vi "Plate Tank 4.vi"() -> ()   [LabVIEW 2019]
uses:
  <vilib>/NI/Current Value Table/Type Defs/Single Tag.ctl
  <vilib>/NI/Current Value Table/Type Defs/Data Types.ctl
  <vilib>/Utility/sysdir.llb/System Directory Type.ctl
  <vilib>/NI/STM/TCP/Read Meta Data (TCP Ref).vi
  <vilib>/NI/STM/TCP/Get Connection Reference (TCP).vi
  <vilib>/NI/AMC/Read Termination Message.vi
  <vilib>/NI/AMC/Create Single Message.vi
  <vilib>/NI/AMC/Update Message Routing Info.vi
  <vilib>/NI/STM/TCP/Read Meta Data (TCP Clst).vi
  <vilib>/NI/AMC/Send Message.vi
  <vilib>/NI/AMC/Globals.vi
  <userlib>/_OpenG.lib/comparison/comparison.llb/I32 Changed__ogtk.vi
  <vilib>/NI/STM/TCP/Write Message (TCP).vi
  <vilib>/NI/AMC/AMC.lvlib
  <vilib>/NI/STM/NI STM.lvlib
  <vilib>/NI/Current Value Table/Current Value Table.lvlib
panel:
  in  "EZ Recipe Button":bool
  out "Loaded Recipe":string
  in  "Load A Recipe":bool
  in  "Save this Recipe":bool
  out "Right Time":dbl format="%.1f"
  out "Left Time":dbl format="%.1f"
  out "Total Amp*min R":dbl format="%.1f"
  out "Total Amp*min L":dbl format="%.1f"
  in  "Rectifer Settings":i32(listbox)
  in  "MO":string
  in  "BasT1_P Last Hr":bool
  in  "BasT1_Level Last Hr":bool
  out "Boolean 5":bool
  out "SumpBottom":bool
  out "Process 1 Supply":bool
  out "Sump Return":bool
  out "Boolean 2":bool
  out "SG":dbl format="%.3g"
  out "Return to sump 4":bool
  in  "Rectifer Data":enum32{"Standard", "Eng"}(tab)
  out "Current Step":i32
  out "Left Anode Actual Current":dbl(knob) scale=0.0..150.0
  out "Right Anode Actual Current":dbl(knob) scale=0.0..150.0
  out "Left Anode Amp-min":dbl(slide)
  out "Right Anode Amp-min":dbl(slide)
  out "Output Voltage":cluster{dbl, dbl}(graph)
  in  "Tab Control 2":enum32{"Standard", "ENG"}(tab)
  out "Supply Flow":dbl(knob) scale=0.0..65.0
  out "Plating Cell Liquid Level":dbl(slide) scale=0.0..75.0
  out "Cell Temperature":dbl(slide) scale=0.0..60.0
  in  "Cell T Last Hr":bool
  out "Suck Pump":bool
  out "Suck Pump Flow":dbl format="%#_4g"
  out "SuckPipe":bool
  out "SuckPipe 3":bool
  out "Drain Tee Top":bool
  out "Return to sump 2":bool
  out "Return to sump 3":bool
  out "Flow Controller":dbl(knob) scale=0.0..100.0
  in  "Tab Control":enum32{"Main Pump", "Suck Pump"}(tab)
  out "Amps":dbl format="%#.2g"
  out "Volts":dbl format="%#.1f"
  out "VFD T":dbl format="%#.2g"
  out "RPM":dbl format="%#.0f"
  out "Fault Code":dbl format="%#.2g"
  out "Freq":dbl format="%#.2g"
  out "SP1 Amps":dbl caption="Amps" format="%#.2g"
  out "SP1 Volts":dbl caption="Volts" format="%#.1g"
  out "SP1 RPM":dbl caption="RPM" format="%#.2g"
  out "SP1 VFD T":dbl caption="VFD T" format="%#.2g"
  out "SP1 Fault Code":dbl caption="Fault Code" format="%#.2g"
  out "SP1 Freq":dbl caption="Freq" format="%#.2g"
  out "Flow 1":dbl format="%#_4g"
  out "Flow 2":dbl format="%#_4g"
  out "Flow 3":dbl format="%#_4g"
  out "Flow 4":dbl format="%#_4g"
  out "Return to sump":bool
  out "E Stop":bool
  out "Run Enabled?":bool
  in  "Full Drain Plating Cell":bool
  out "Rack Motion":bool
  out "Right Eductor Motion":bool
  out "Left Eductor Motion":bool
  out "Right Output On":bool
  in  "Enable Rack Motion":bool
  in  "Rack RPM":dbl(knob) scale=0.0..15.0
  out "Left Output On":bool
  in  "Start Cycle":bool
  in  "Cancel Cycle":bool
  out "SuckPipe 2":bool
  out "Main Pump":bool
  in  "Enable Eductor Motion":bool
  in  "Eductor RPM":dbl(knob) scale=0.0..15.0
  in  "Supply Pressure (kPa)":dbl(knob)=50.0 min=50.0 max=200.0 step=5.0 scale=50.0..200.0
  in  "Total Inflow (L/min)":dbl(knob)=40.0 min=25.0 max=50.0 step=0.5 scale=25.0..50.0
  in  "Suck Pump fraction of inflow":dbl(knob)=5.0 min=5.0 max=90.0 step=1.0 scale=0.0..90.0
  out "Sump Level":dbl(slide) scale=0.0..1000.0
  out "Supply Pressure":dbl(knob) scale=0.0..200.0
  in  "Enable Suck Pump":bool
  in  "Enable Plating Cell":bool
  in  "Machine":bool
  in  "Basement 4":bool
  in  "Dryer":bool
  in  "Rinse 4":bool
  in  "Rinse 3":bool
  in  "Rinse 2":bool
  in  "Basement 3":bool
  in  "Basement 2":bool
  in  "Basement 1":bool
  in  "Plater 6":bool
  in  "Plater 5":bool
  in  "Plater 4":bool
  in  "Plater 3":bool
  in  "Plater 2":bool
  in  "Plater 1":bool
  in  "Predip":bool
  in  "Rinse 1":bool
  in  "Cleaner":bool
  in  "Etch":bool
  out "status":string
  out "Boolean 4":bool
  # "Module Selection"
  # "Rectifier Settings"
  # "Recipe"
  # "Fluid Flow Control"
  # "Rectifier Control"
  # "Rectifier Output"
  # "Motion starts when rectifiers cycle"
  # "Note: RPM settings shared with tank 4"
  # "kPa"
  # "@"
  # "Output"
  # "cm"
  # "°C"
  # "L/min"
  # "cm"
  # "L/min"
  # "L/min"
  # "L/min"
  # "L/min"
  # "L/min"
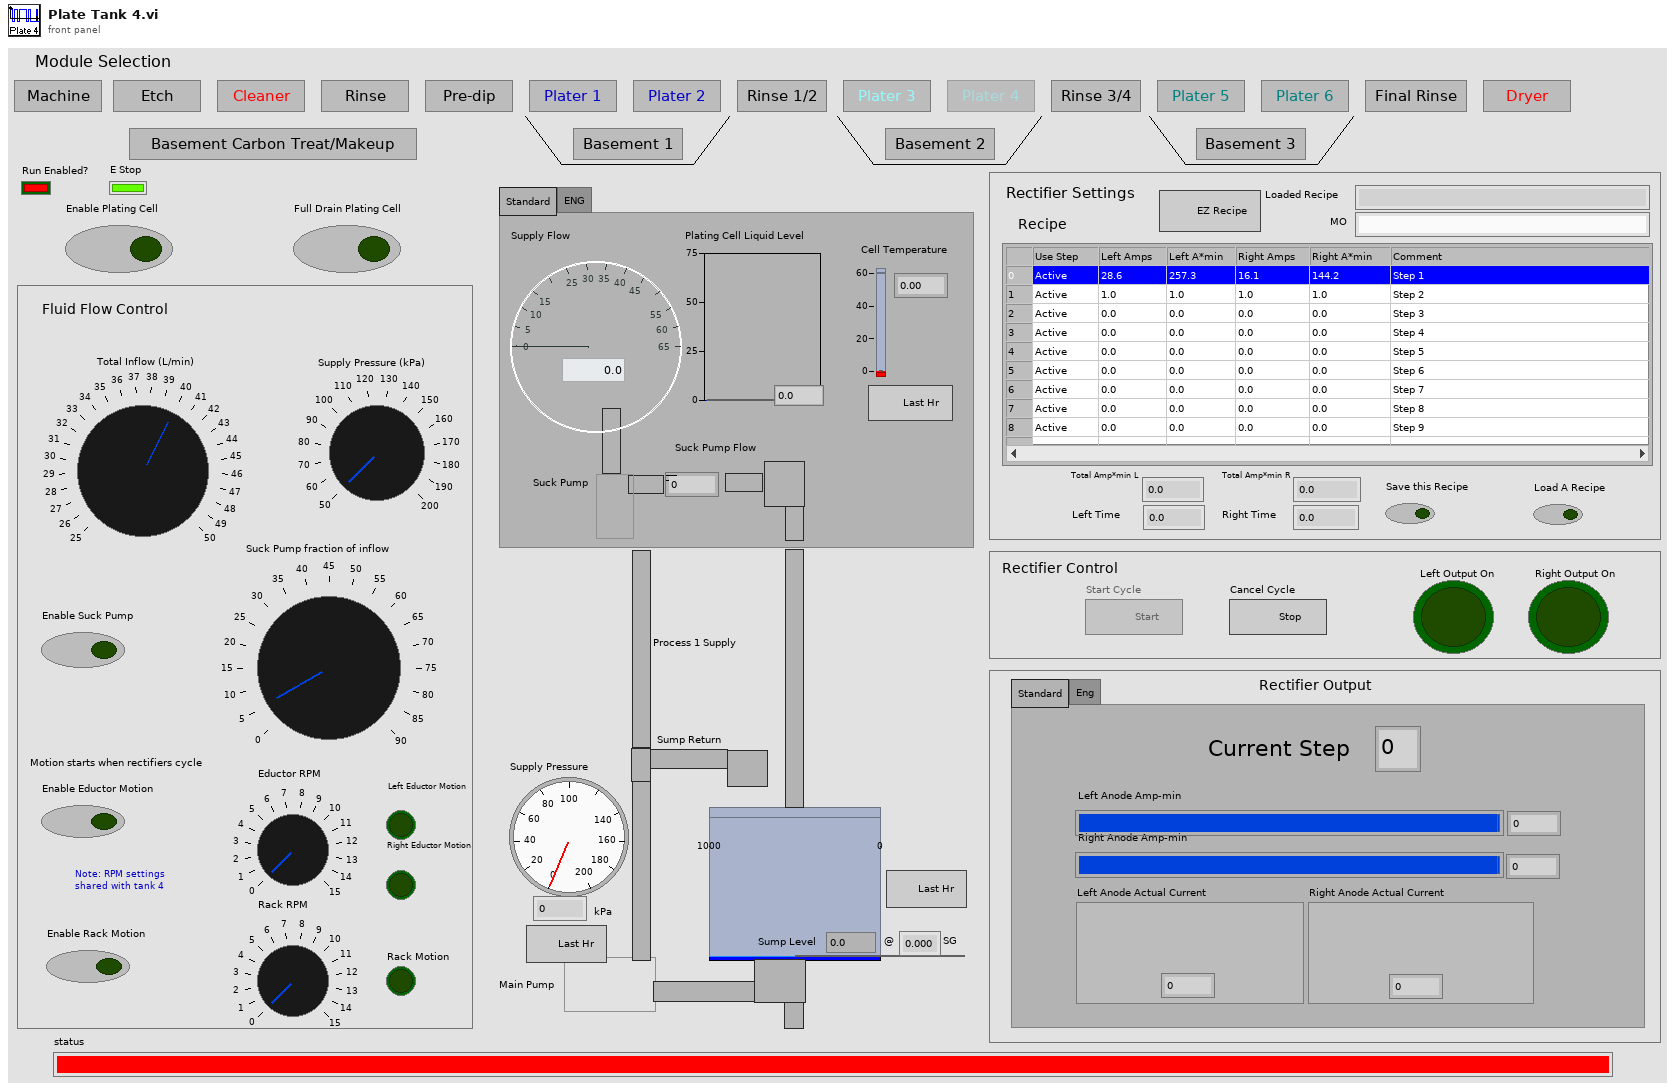
[diagram p1: front panel]
types:
  T1 = typedef "Current Value Table.lvlib/Single Tag.ctl" = cluster{"Data Type":T2, "Name":string, "Value":string, "Description":string}
  T2 = typedef "Current Value Table.lvlib/Data Types.ctl" = enum16{"Double", "Single", "I64", "I32", "I16", "I8", "U64", "U32", "U16", "U8", "String", "Boolean", "Array of U8", "Array of U16", "Array of U32", "Array of U64", "Array of I64", "Array of I32", "Array of I16", "Array of I8", "Array of Double", "Array of Single", "Array of Boolean", "Array of String"}
  T3 = typedef "NI STM.lvlib/TCP Connection Info.ctl" = cluster{"connection ID":refnum<k5>, "meta data":T4[]}
  T4 = typedef "NI STM.lvlib/MetaDataElement.ctl" = string
  T5 = typedef "AMC.lvlib/Message Queue.ctl" = refnum<queue>
  T6 = cluster{"Shift":bool, "Ctrl":bool, "Alt":bool, "Cmd":bool, "Opt":bool}
  T7 = typedef "LVPoint32TypeDef.ctl" = cluster{"Horizontal":i32, "Vertical":i32}
  T8 = typedef "LVRowAndColumnTypeDef.ctl" = cluster{"Row":i32, "Column":i32}
  T9 = enum8{"Enabled", "Disabled", "Disabled and Grayed Out"}
  T10 = typedef "System Directory Type.ctl" = i32
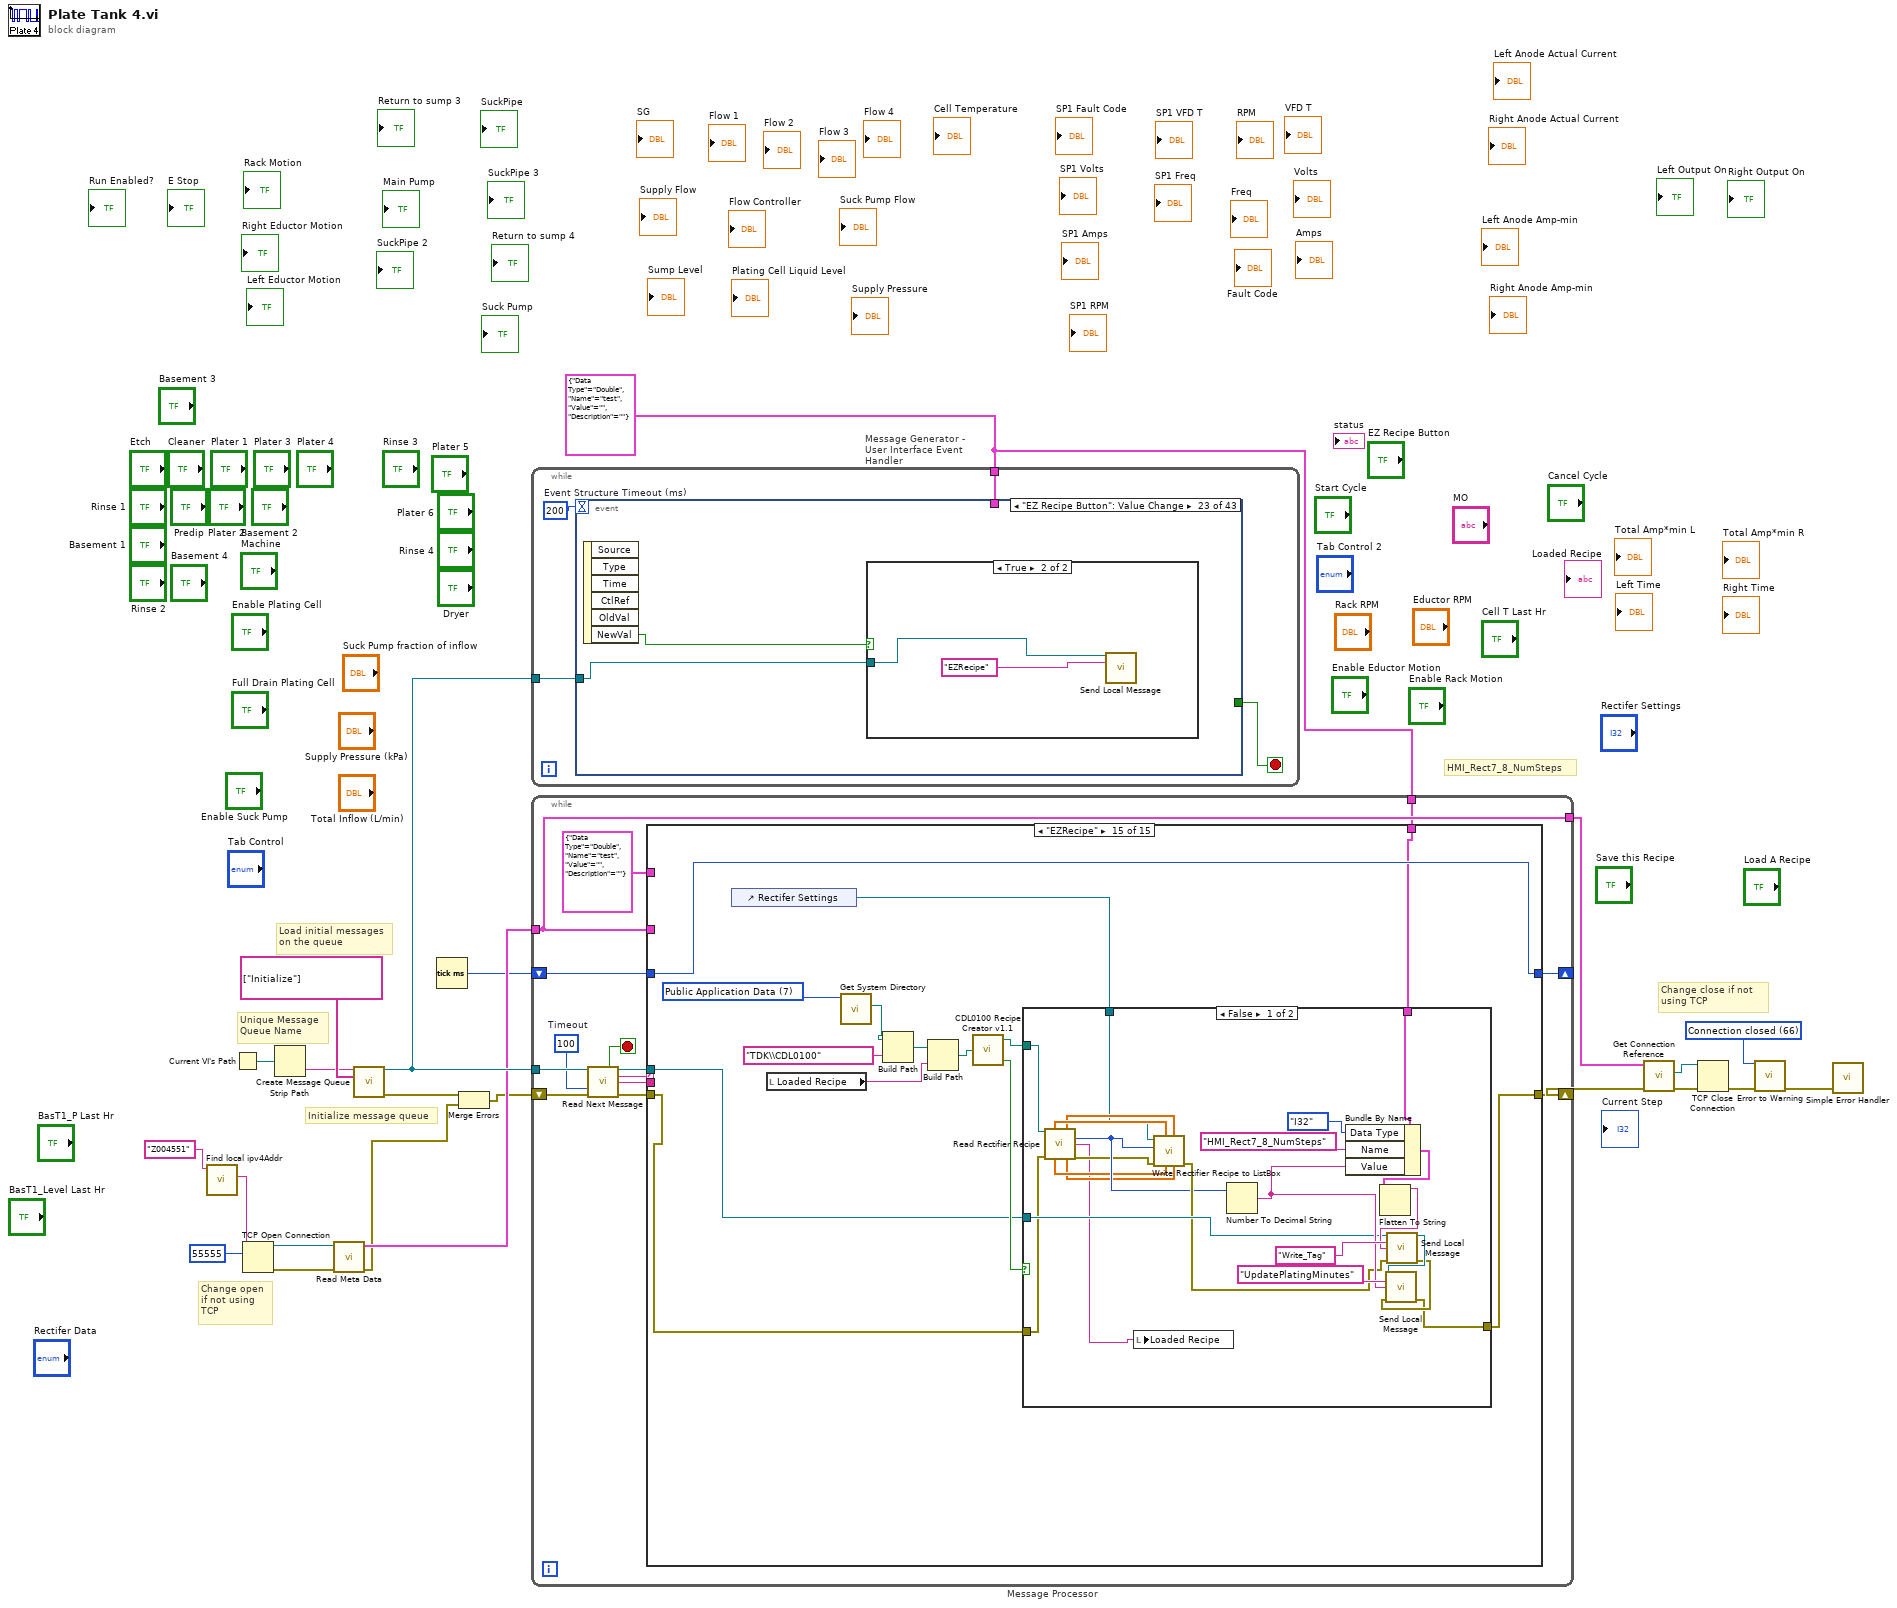
[diagram p0: block diagram]
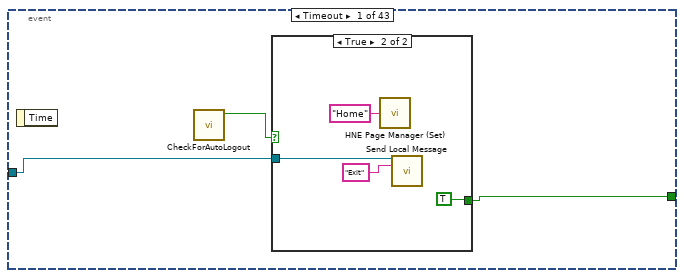
[diagram p2: hidden frame]
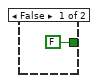
[diagram p3: hidden frame]
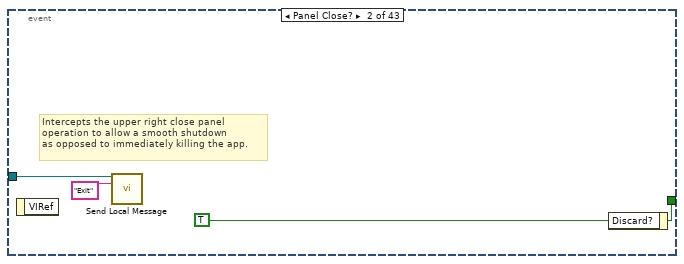
[diagram p4: hidden frame]
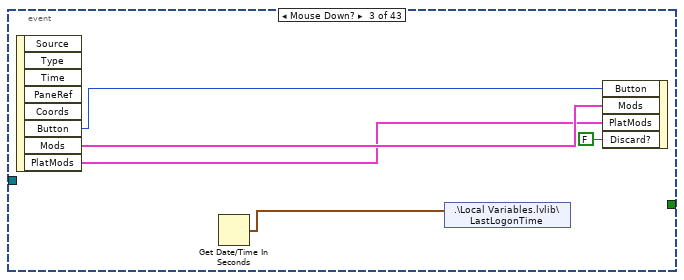
[diagram p5: hidden frame]
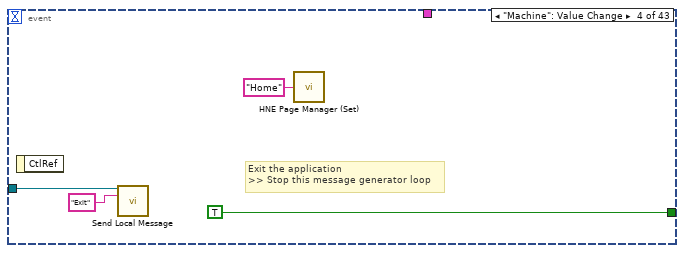
[diagram p6: hidden frame]
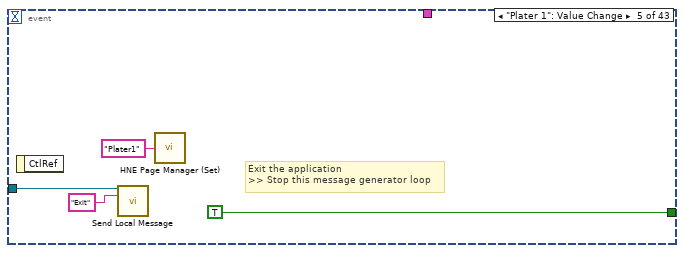
[diagram p7: hidden frame]
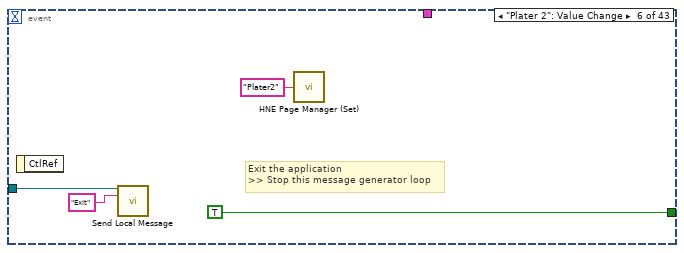
[diagram p8: hidden frame]
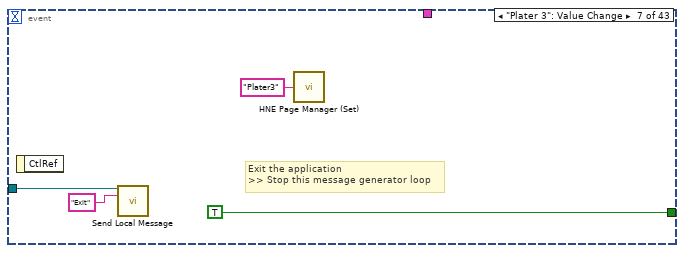
[diagram p9: hidden frame]
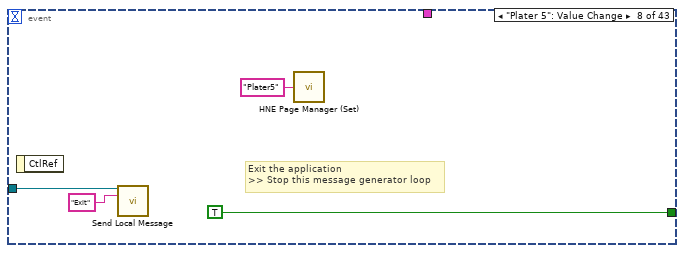
[diagram p10: hidden frame]
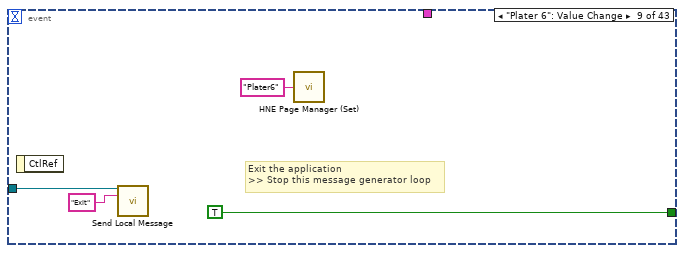
[diagram p11: hidden frame]
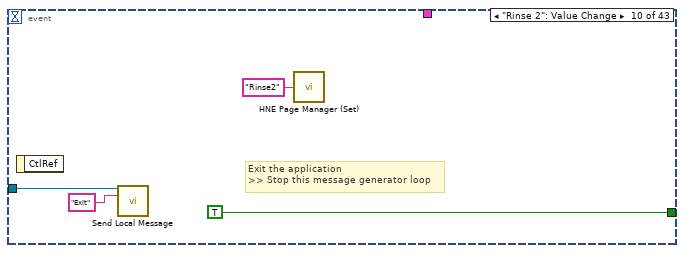
[diagram p12: hidden frame]
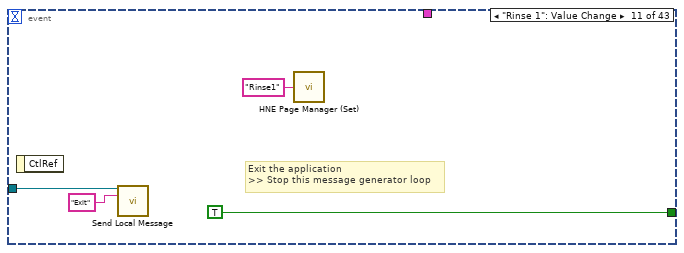
[diagram p13: hidden frame]
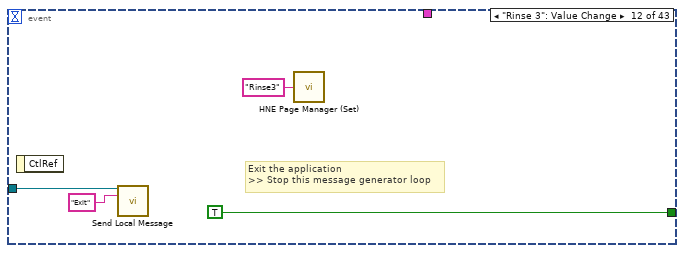
[diagram p14: hidden frame]
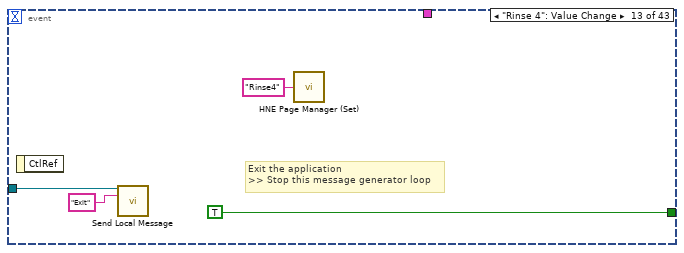
[diagram p15: hidden frame]
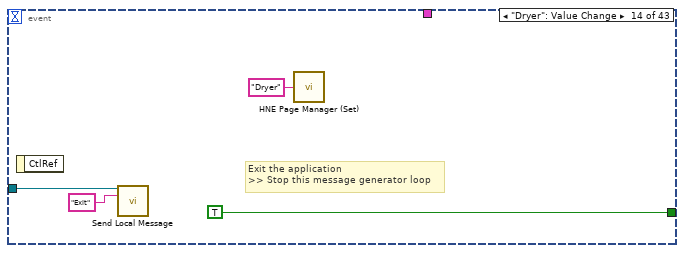
[diagram p16: hidden frame]
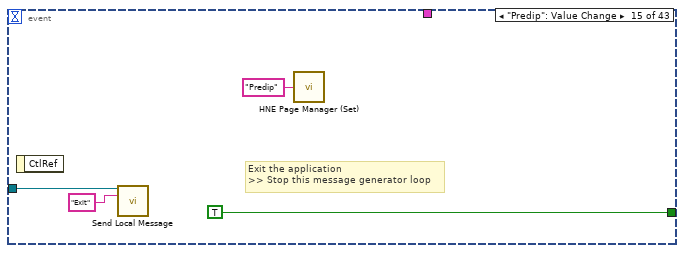
[diagram p17: hidden frame]
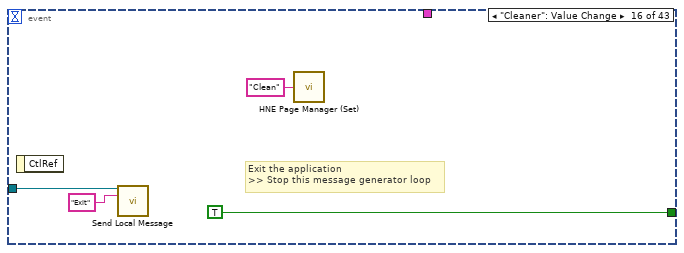
[diagram p18: hidden frame]
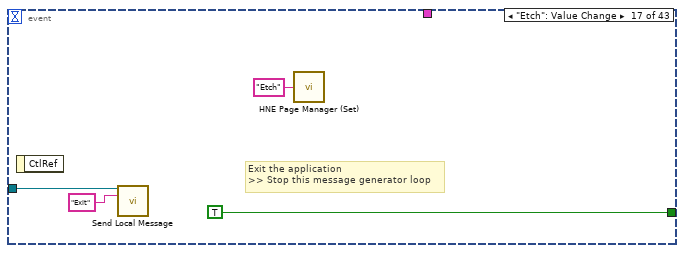
[diagram p19: hidden frame]
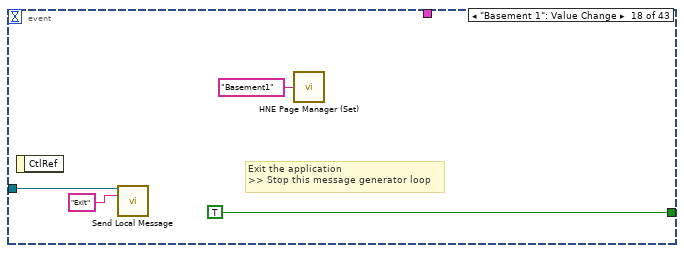
[diagram p20: hidden frame]
diagram:
  w1 = T1 {"Data Type"=enum."Double", "Name"="test", "Value"="", "Description"=""} ("Tag")
  w13 = 66 items=["No Error", "Argument Error", "Memory Full", "Out of Zone", "End of File", "File Already Open", "Generic File IO Error", "File Not Found", "File Permission Error", "Disk Full", "Duplicate Path", "Too Many Files Open", "Not Enabled", "Resource File Not Found", "Cannot Add Resource", "Resource Not Found", "Image Not Found", "Image Memory Error", "Pen Does Not Exist", "Config Bad Type", "Config Token Not Found", "Config Parse Error", "Config Memory Error", "Bad External Code Format", "Bad External Code Offset", "External Code Not Present", "Null Window", "Destroy Window Mixup", "Null Menu", "Print Aborted", "Bad Print Record", "Print Driver Error", "Windows Error During Print", "Memory Error During Print", "Print Dialog Error", "Generic Print Error", "Invalid Device Refnum", "Device Not Found", "Device Parameter Error", "Device Unit Error", "Can't Open Device", "Device Call Aborted", "Generic Error", "Cancelled By User", "Object ID Too Low", "Object ID Too High", "Object Not In Heap", "Unknown Heap", "Bad DefProc ID", "DefProc Not In Table", "Message Out Of Range", "Null Method", "Unknown Message", "Manager Call Not Supported", "Bad address", "Connection In progress", "Connection timed out", "Connection is already in progress", "Network attribute not supported", "Network error", "Address in use", "System out of memory", "Connection aborted", "Connection refused", "Connection is not connected", "Connection is already connected", "Connection closed", "Initialize error (interapplication manager)", "Bad occurrence", "Wait on unbound occurrence handler", "Occurrence queue overflow", "Bad path", "Semaphore not signaled", "Unrecognized type (interapplication manager)"] ("1st Error to Convert")
  # "HMI_Rect7_8_NumSteps"
  # "Change close if not using TCP"
  # "Change open if not using TCP"
  # "Initialize message queue"
  # "Unique Message\nQueue Name"
  # "Load initial messages\non the queue"
  n1 = call "Find local ipv4Addr.vi"("MachineToFind"="Z004551" ("Target IP Address")) -> ("name"=w5:string)  [unwired: 9 in, 1 out]
  n2 = Current VI's Path() -> (path=w19:path)
  n3 = TCP Open Connection(address=w5, remote port or service name=u16 55555 ("remote port")) -> (connection ID=w17:refnum<k5>, error out=w16:errorcluster)  [unwired: 1 in, 2 out]
  n4 = Strip Path(path=w19) -> (name=w21:string)  [unwired: 1 out]
  n5 = call-poly <vilib>:"Read Meta Data.vi"("error in"=w16, "connection ID"=w17) -> ("error out"=w3:errorcluster, "connection info out"=w15:T3)  [unwired: 7 in, 1 out]
  n6 = call <vilib>:"Create Message Queue.vi"("message queue name"=w21, "initial message names"=string[] ["Initialize"]) -> ("message queue out"=w20:T5, "error out"=w4:errorcluster)  [unwired: 12 in]
  n7 = Tick Count (ms)() -> (millisecond timer value=w7:u32)
  n8 = Merge Errors(w4, w3) -> (w2:errorcluster)
  n9 = while "Message Generator - User Interface Event Handler" {
    tunnel: w20 -> [w24]
    tunnel: w1 -> [w23]
    stop <- w25 stop-if-true
    w26 = 200  # Event Structure Timeout (ms)
    n10 = event shown="[22] \"EZ Recipe Button\": Value Change" {
      selector: _ -> [_ _ _ _ _ _ _ _ _ _ _ _ _ _ _ _ _ _ _ _ _ _ _ _ _ _ _ _ _ _ _ _ _ _ _ _ _ _ _ _ _ _ _]
      dyn-events: _ -> [_ _ _ _ _ _ _ _ _ _ _ _ _ _ _ _ _ _ _ _ _ _ _ _ _ _ _ _ _ _ _ _ _ _ _ _ _ _ _ _ _ _ _]
      timeout: w26 -> [_ _ _ _ _ _ _ _ _ _ _ _ _ _ _ _ _ _ _ _ _ _ _ _ _ _ _ _ _ _ _ _ _ _ _ _ _ _ _ _ _ _ _]
      tunnel: [w27 w37 _ TRUE ("Discard?") TRUE ("Discard?") TRUE ("Discard?") TRUE ("Discard?") TRUE ("Discard?") TRUE ("Discard?") TRUE ("Discard?") TRUE ("Discard?") TRUE ("Discard?") TRUE ("Discard?") TRUE ("Discard?") TRUE ("Discard?") TRUE ("Discard?") TRUE ("Discard?") TRUE ("Discard?") TRUE ("Discard?") TRUE ("Discard?") TRUE ("Discard?") FALSE ("Discard?") _ FALSE ("Discard?") FALSE ("Discard?") FALSE ("Discard?") FALSE ("Discard?") FALSE ("Discard?") FALSE ("Discard?") FALSE ("Discard?") FALSE ("Discard?") FALSE ("Discard?") FALSE ("Discard?") FALSE ("Discard?") FALSE ("Discard?") FALSE ("Discard?") _ _ _ _ _ _ _] -> w25
      tunnel: w24 -> [w28 w35 _ w44 w48 w52 w56 w60 w64 w68 w72 w76 w80 w84 w88 w92 w96 w100 w104 w108 w112 w118 w121 w125 w130 w143 w154 w165 w176 w180 w194 w214 w224 w234 w244 w256 w258 w260 w265 w270 _ w277 w299]
      tunnel: w23 -> [_ _ _ _ _ _ _ _ _ _ _ _ _ _ _ _ _ _ _ _ _ _ _ _ _ w140 w151 w162 w173 w179 w193 w213 w223 w233 w243 w255 _ _ _ _ _ w276 _]
      event Timeout {
        n11 = event-data() -> ()  [unwired: 2 out]
        n12 = call "CheckForAutoLogout.vi"() -> ("Boolean"=w29:bool)  [unwired: 11 in]
        n13 = case shown="True" w29 {
          tunnel: [FALSE ("Discard?") TRUE ("Discard?")] -> w27
          tunnel: w28 -> [_ w31]
          frame False {
          }
          frame True {
            n14 = call <userlib>:"HNE Page Manager (Set).vi"("Next Page"="Home") -> ()  [unwired: 4 in, 1 out]
            n15 = call <vilib>:"Send Local Message.vi"("message queue in"=w31, "message name"="Exit") -> ()  [unwired: 11 in, 3 out]
          }
        }
      }
      event Panel Close? {
        w37 = TRUE ("Discard?")
        # "Intercepts the upper right close panel\noperation to allow a smooth shutdown\nas opposed to immediately killing the app."
        n16 = event-data() -> ()  [unwired: 2 out]
        n17 = call <vilib>:"Send Local Message.vi"("message queue in"=w35, "message name"="Exit") -> ()  [unwired: 11 in, 3 out]
        n18 = event-data("Discard?"=w37) -> ()  [unwired: 1 in, 1 out]
      }
      event Mouse Down? {
        n19 = event-data() -> ("Button"=w42:u16, "Mods"=w40:cluster{"Double Click":bool, "Menu Key":bool}, "PlatMods"=w39:T6)  [unwired: 6 out]
        n20 = Get Date/Time In Seconds() -> (seconds since 1Jan1904=w38:timestamp)
        n21 = shared-variable ".\\Local Variables.lvlib\\LastLogonTime"(w38) -> ()  [unwired: 1 in, 1 out]
        n22 = event-data("Button"=w42, "Mods"=w40, "PlatMods"=w39, "Discard?"=FALSE) -> ()  [unwired: 1 in, 1 out]
      }
      event "Machine": Value Change {
        # "Exit the application\n>> Stop this message generator loop"
        n23 = event-data() -> ()  [unwired: 2 out]
        n24 = call <vilib>:"Send Local Message.vi"("message queue in"=w44, "message name"="Exit") -> ()  [unwired: 11 in, 3 out]
        n25 = call <userlib>:"HNE Page Manager (Set).vi"("Next Page"="Home") -> ()  [unwired: 4 in, 1 out]
      }
      event "Plater 1": Value Change {
        # "Exit the application\n>> Stop this message generator loop"
        n26 = event-data() -> ()  [unwired: 2 out]
        n27 = call <vilib>:"Send Local Message.vi"("message queue in"=w48, "message name"="Exit") -> ()  [unwired: 11 in, 3 out]
        n28 = call <userlib>:"HNE Page Manager (Set).vi"("Next Page"="Plater1") -> ()  [unwired: 4 in, 1 out]
      }
      event "Plater 2": Value Change {
        # "Exit the application\n>> Stop this message generator loop"
        n29 = event-data() -> ()  [unwired: 2 out]
        n30 = call <vilib>:"Send Local Message.vi"("message queue in"=w52, "message name"="Exit") -> ()  [unwired: 11 in, 3 out]
        n31 = call <userlib>:"HNE Page Manager (Set).vi"("Next Page"="Plater2") -> ()  [unwired: 4 in, 1 out]
      }
      event "Plater 3": Value Change {
        # "Exit the application\n>> Stop this message generator loop"
        n32 = event-data() -> ()  [unwired: 2 out]
        n33 = call <vilib>:"Send Local Message.vi"("message queue in"=w56, "message name"="Exit") -> ()  [unwired: 11 in, 3 out]
        n34 = call <userlib>:"HNE Page Manager (Set).vi"("Next Page"="Plater3") -> ()  [unwired: 4 in, 1 out]
      }
      event "Plater 5": Value Change {
        # "Exit the application\n>> Stop this message generator loop"
        n35 = event-data() -> ()  [unwired: 2 out]
        n36 = call <vilib>:"Send Local Message.vi"("message queue in"=w60, "message name"="Exit") -> ()  [unwired: 11 in, 3 out]
        n37 = call <userlib>:"HNE Page Manager (Set).vi"("Next Page"="Plater5") -> ()  [unwired: 4 in, 1 out]
      }
      event "Plater 6": Value Change {
        # "Exit the application\n>> Stop this message generator loop"
        n38 = event-data() -> ()  [unwired: 2 out]
        n39 = call <vilib>:"Send Local Message.vi"("message queue in"=w64, "message name"="Exit") -> ()  [unwired: 11 in, 3 out]
        n40 = call <userlib>:"HNE Page Manager (Set).vi"("Next Page"="Plater6") -> ()  [unwired: 4 in, 1 out]
      }
      event "Rinse 2": Value Change {
        # "Exit the application\n>> Stop this message generator loop"
        n41 = event-data() -> ()  [unwired: 2 out]
        n42 = call <vilib>:"Send Local Message.vi"("message queue in"=w68, "message name"="Exit") -> ()  [unwired: 11 in, 3 out]
        n43 = call <userlib>:"HNE Page Manager (Set).vi"("Next Page"="Rinse2") -> ()  [unwired: 4 in, 1 out]
      }
      event "Rinse 1": Value Change {
        # "Exit the application\n>> Stop this message generator loop"
        n44 = event-data() -> ()  [unwired: 2 out]
        n45 = call <vilib>:"Send Local Message.vi"("message queue in"=w72, "message name"="Exit") -> ()  [unwired: 11 in, 3 out]
        n46 = call <userlib>:"HNE Page Manager (Set).vi"("Next Page"="Rinse1") -> ()  [unwired: 4 in, 1 out]
      }
      event "Rinse 3": Value Change {
        # "Exit the application\n>> Stop this message generator loop"
        n47 = event-data() -> ()  [unwired: 2 out]
        n48 = call <vilib>:"Send Local Message.vi"("message queue in"=w76, "message name"="Exit") -> ()  [unwired: 11 in, 3 out]
        n49 = call <userlib>:"HNE Page Manager (Set).vi"("Next Page"="Rinse3") -> ()  [unwired: 4 in, 1 out]
      }
      event "Rinse 4": Value Change {
        # "Exit the application\n>> Stop this message generator loop"
        n50 = event-data() -> ()  [unwired: 2 out]
        n51 = call <vilib>:"Send Local Message.vi"("message queue in"=w80, "message name"="Exit") -> ()  [unwired: 11 in, 3 out]
        n52 = call <userlib>:"HNE Page Manager (Set).vi"("Next Page"="Rinse4") -> ()  [unwired: 4 in, 1 out]
      }
      event "Dryer": Value Change {
        # "Exit the application\n>> Stop this message generator loop"
        n53 = event-data() -> ()  [unwired: 2 out]
        n54 = call <vilib>:"Send Local Message.vi"("message queue in"=w84, "message name"="Exit") -> ()  [unwired: 11 in, 3 out]
        n55 = call <userlib>:"HNE Page Manager (Set).vi"("Next Page"="Dryer") -> ()  [unwired: 4 in, 1 out]
      }
      event "Predip": Value Change {
        # "Exit the application\n>> Stop this message generator loop"
        n56 = event-data() -> ()  [unwired: 2 out]
        n57 = call <vilib>:"Send Local Message.vi"("message queue in"=w88, "message name"="Exit") -> ()  [unwired: 11 in, 3 out]
        n58 = call <userlib>:"HNE Page Manager (Set).vi"("Next Page"="Predip") -> ()  [unwired: 4 in, 1 out]
      }
      event "Cleaner": Value Change {
        # "Exit the application\n>> Stop this message generator loop"
        n59 = event-data() -> ()  [unwired: 2 out]
        n60 = call <vilib>:"Send Local Message.vi"("message queue in"=w92, "message name"="Exit") -> ()  [unwired: 11 in, 3 out]
        n61 = call <userlib>:"HNE Page Manager (Set).vi"("Next Page"="Clean") -> ()  [unwired: 4 in, 1 out]
      }
      event "Etch": Value Change {
        # "Exit the application\n>> Stop this message generator loop"
        n62 = event-data() -> ()  [unwired: 2 out]
        n63 = call <vilib>:"Send Local Message.vi"("message queue in"=w96, "message name"="Exit") -> ()  [unwired: 11 in, 3 out]
        n64 = call <userlib>:"HNE Page Manager (Set).vi"("Next Page"="Etch") -> ()  [unwired: 4 in, 1 out]
      }
      event "Basement 1": Value Change {
        # "Exit the application\n>> Stop this message generator loop"
        n65 = event-data() -> ()  [unwired: 2 out]
        n66 = call <vilib>:"Send Local Message.vi"("message queue in"=w100, "message name"="Exit") -> ()  [unwired: 11 in, 3 out]
        n67 = call <userlib>:"HNE Page Manager (Set).vi"("Next Page"="Basement1") -> ()  [unwired: 4 in, 1 out]
      }
      event "Basement 2": Value Change {
        # "Exit the application\n>> Stop this message generator loop"
        n68 = event-data() -> ()  [unwired: 2 out]
        n69 = call <vilib>:"Send Local Message.vi"("message queue in"=w104, "message name"="Exit") -> ()  [unwired: 11 in, 3 out]
        n70 = call <userlib>:"HNE Page Manager (Set).vi"("Next Page"="Basement2") -> ()  [unwired: 4 in, 1 out]
      }
      event "Basement 3": Value Change {
        # "Exit the application\n>> Stop this message generator loop"
        n71 = event-data() -> ()  [unwired: 2 out]
        n72 = call <vilib>:"Send Local Message.vi"("message queue in"=w108, "message name"="Exit") -> ()  [unwired: 11 in, 3 out]
        n73 = call <userlib>:"HNE Page Manager (Set).vi"("Next Page"="Basement3") -> ()  [unwired: 4 in, 1 out]
      }
      event "Basement 4": Value Change {
        # "Exit the application\n>> Stop this message generator loop"
        n74 = event-data() -> ()  [unwired: 2 out]
        n75 = call <vilib>:"Send Local Message.vi"("message queue in"=w112, "message name"="Exit") -> ()  [unwired: 11 in, 3 out]
        n76 = call <userlib>:"HNE Page Manager (Set).vi"("Next Page"="Basement4") -> ()  [unwired: 4 in, 1 out]
      }
      event "Enable Plating Cell": Value Change {
        n77 = event-data() -> ("NewVal"=w116:bool)  [unwired: 1 out]
        n78 = call "Validate Plate Tank Enable.vi"("Valve No."=144, "Test Value"=w116, "Tag"="HMI_Tank4_Enable", "Queue in"=w118) -> ()  [unwired: 8 in]
      }
      event "EZ Recipe Button": Value Change {
        n79 = event-data() -> ("NewVal"=w120:bool)  [unwired: 6 out]
        n80 = case shown="True" w120 {
          tunnel: w121 -> [_ w122]
          frame False {
          }
          frame True {
            n81 = call <vilib>:"Send Local Message.vi"("message queue in"=w122, "message name"="EZRecipe") -> ()  [unwired: 11 in, 3 out]
          }
        }
      }
      event "Save this Recipe": Value Change {
        n82 = event-data() -> ("NewVal"=w124:bool)  [unwired: 1 out]
        n83 = case shown="True" w124 {
          tunnel: w125 -> [_ w128]
          frame False {
          }
          frame True {
            n84 = call <vilib>:"Send Local Message.vi"("message queue in"=w128, "message name"="Save_Recipe") -> ()  [unwired: 11 in, 3 out]
          }
        }
      }
      event "Load A Recipe": Value Change {
        n85 = event-data() -> ("NewVal"=w129:bool)  [unwired: 1 out]
        n86 = case shown="True" w129 {
          tunnel: w130 -> [_ w133]
          frame False {
          }
          frame True {
            n87 = call <vilib>:"Send Local Message.vi"("message queue in"=w133, "message name"="Load_A_Recipe") -> ()  [unwired: 11 in, 3 out]
          }
        }
      }
      event "Full Drain Plating Cell": Value Change {
        n88 = event-data() -> ("NewVal"=w142:bool)  [unwired: 1 out]
        n89 = Boolean To (0,1)(Boolean=w142) -> (0, 1=w141:i16)
        n90 = Number To Decimal String(number=w141) -> (decimal integer string=w137:string)  [unwired: 1 in]
        n91 = Bundle By Name(cluster=w140, "Data Type"=Data_Types."Boolean", "Name"="HMI_Tank4_Drain", "Value"=w137) -> (w136:T1)
        n92 = Flatten To String(anything=w136) -> (data string=w135:string)  [unwired: 3 in, 2 out]
        n93 = call <vilib>:"Send Local Message.vi"("message queue in"=w143, "message name"="Write_Tag", "message value"=w135) -> ()  [unwired: 10 in, 3 out]
      }
      event "Enable Eductor Motion": Value Change {
        n94 = event-data() -> ("NewVal"=w153:bool)  [unwired: 1 out]
        n95 = Boolean To (0,1)(Boolean=w153) -> (0, 1=w152:i16)
        n96 = Number To Decimal String(number=w152) -> (decimal integer string=w148:string)  [unwired: 1 in]
        n97 = Bundle By Name(cluster=w151, "Data Type"=Data_Types."Boolean", "Name"="HMI_Tank4_Eductor_Motors_Run", "Value"=w148) -> (w147:T1)
        n98 = Flatten To String(anything=w147) -> (data string=w146:string)  [unwired: 3 in, 2 out]
        n99 = call <vilib>:"Send Local Message.vi"("message queue in"=w154, "message name"="Write_Tag", "message value"=w146) -> ()  [unwired: 10 in, 3 out]
      }
      event "Enable Rack Motion": Value Change {
        n100 = event-data() -> ("NewVal"=w164:bool)  [unwired: 1 out]
        n101 = Boolean To (0,1)(Boolean=w164) -> (0, 1=w163:i16)
        n102 = Number To Decimal String(number=w163) -> (decimal integer string=w159:string)  [unwired: 1 in]
        n103 = Bundle By Name(cluster=w162, "Data Type"=Data_Types."Boolean", "Name"="HMI_Tank4_Rack_Motor_Run", "Value"=w159) -> (w158:T1)
        n104 = Flatten To String(anything=w158) -> (data string=w157:string)  [unwired: 3 in, 2 out]
        n105 = call <vilib>:"Send Local Message.vi"("message queue in"=w165, "message name"="Write_Tag", "message value"=w157) -> ()  [unwired: 10 in, 3 out]
      }
      event "Enable Suck Pump": Value Change {
        n106 = event-data() -> ("NewVal"=w175:bool)  [unwired: 1 out]
        n107 = Boolean To (0,1)(Boolean=w175) -> (0, 1=w174:i16)
        n108 = Number To Decimal String(number=w174) -> (decimal integer string=w170:string)  [unwired: 1 in]
        n109 = Bundle By Name(cluster=w173, "Data Type"=Data_Types."Boolean", "Name"="HMI_Tnk4_Enable_SuckPump", "Value"=w170) -> (w169:T1)
        n110 = Flatten To String(anything=w169) -> (data string=w168:string)  [unwired: 3 in, 2 out]
        n111 = call <vilib>:"Send Local Message.vi"("message queue in"=w176, "message name"="Write_Tag", "message value"=w168) -> ()  [unwired: 10 in, 3 out]
      }
      event "Start Cycle": Value Change {
        n112 = event-data() -> ("NewVal"=w178:bool)  [unwired: 1 out]
        n113 = case shown="True" w178 {
          tunnel: w180 -> [_ w191]
          tunnel: w178 -> [_ w190]
          tunnel: w179 -> [_ w188]
          frame False {
          }
          frame True {
            n114 = Boolean To (0,1)(Boolean=w190) -> (0, 1=w189:i16)
            n115 = Number To Decimal String(number=w189) -> (decimal integer string=w185:string)  [unwired: 1 in]
            n116 = Bundle By Name(cluster=w188, "Data Type"=Data_Types."Boolean", "Name"="HMI_Rect7_8_Cycle", "Value"=w185) -> (w184:T1)
            n117 = Flatten To String(anything=w184) -> (data string=w183:string)  [unwired: 3 in, 2 out]
            n118 = call <vilib>:"Send Local Message.vi"("message queue in"=w191, "message name"="Write_Tag", "message value"=w183) -> ()  [unwired: 10 in, 3 out]
          }
        }
      }
      event "Cancel Cycle": Value Change {
        n119 = event-data() -> ("NewVal"=w192:bool)  [unwired: 1 out]
        n120 = case shown="True" w192 {
          tunnel: w194 -> [_ w205]
          tunnel: w192 -> [_ w204]
          tunnel: w193 -> [_ w202]
          frame False {
          }
          frame True {
            n121 = Boolean To (0,1)(Boolean=w204) -> (0, 1=w203:i16)
            n122 = Number To Decimal String(number=w203) -> (decimal integer string=w199:string)  [unwired: 1 in]
            n123 = Bundle By Name(cluster=w202, "Data Type"=Data_Types."Boolean", "Name"="HMI_Rect7_8_CycleStop", "Value"=w199) -> (w198:T1)
            n124 = Flatten To String(anything=w198) -> (data string=w197:string)  [unwired: 3 in, 2 out]
            n125 = call <vilib>:"Send Local Message.vi"("message queue in"=w205, "message name"="Write_Tag", "message value"=w197) -> ()  [unwired: 10 in, 3 out]
          }
        }
      }
      event "Eductor RPM": Value Change {
        n126 = event-data() -> ("NewVal"=w207:dbl)  [unwired: 1 out]
        n127 = Number To Fractional String(number=w207) -> (F-format string=w206:string)  [unwired: 3 in]
        n128 = Bundle By Name(cluster=w213, "Data Type"=Data_Types."Double", "Name"="HMI_Tnk3_Eductor_RPM", "Value"=w206) -> (w210:T1)
        n129 = Flatten To String(anything=w210) -> (data string=w209:string)  [unwired: 3 in, 2 out]
        n130 = call <vilib>:"Send Local Message.vi"("message queue in"=w214, "message name"="Write_Tag", "message value"=w209) -> ()  [unwired: 10 in, 3 out]
      }
      event "Rack RPM": Value Change {
        n131 = event-data() -> ("NewVal"=w217:dbl)  [unwired: 1 out]
        n132 = Number To Fractional String(number=w217) -> (F-format string=w216:string)  [unwired: 3 in]
        n133 = Bundle By Name(cluster=w223, "Data Type"=Data_Types."Double", "Name"="HMI_Tnk3_Rack_RPM", "Value"=w216) -> (w220:T1)
        n134 = Flatten To String(anything=w220) -> (data string=w219:string)  [unwired: 3 in, 2 out]
        n135 = call <vilib>:"Send Local Message.vi"("message queue in"=w224, "message name"="Write_Tag", "message value"=w219) -> ()  [unwired: 10 in, 3 out]
      }
      event "Total Inflow (L/min)": Value Change {
        n136 = event-data() -> ("NewVal"=w227:dbl)  [unwired: 1 out]
        n137 = Number To Fractional String(number=w227) -> (F-format string=w226:string)  [unwired: 3 in]
        n138 = Bundle By Name(cluster=w233, "Data Type"=Data_Types."Double", "Name"="HMI_TNK4_Flow_Setpoint", "Value"=w226) -> (w230:T1)
        n139 = Flatten To String(anything=w230) -> (data string=w229:string)  [unwired: 3 in, 2 out]
        n140 = call <vilib>:"Send Local Message.vi"("message queue in"=w234, "message name"="Write_Tag", "message value"=w229) -> ()  [unwired: 10 in, 3 out]
      }
      event "Supply Pressure (kPa)": Value Change {
        n141 = event-data() -> ("NewVal"=w237:dbl)  [unwired: 1 out]
        n142 = Number To Fractional String(number=w237) -> (F-format string=w236:string)  [unwired: 3 in]
        n143 = Bundle By Name(cluster=w243, "Data Type"=Data_Types."Double", "Name"="HMI_BAS_TNK2_P_Setpoint", "Value"=w236) -> (w240:T1)
        n144 = Flatten To String(anything=w240) -> (data string=w239:string)  [unwired: 3 in, 2 out]
        n145 = call <vilib>:"Send Local Message.vi"("message queue in"=w244, "message name"="Write_Tag", "message value"=w239) -> ()  [unwired: 10 in, 3 out]
      }
      event "Suck Pump fraction of inflow": Value Change {
        n146 = event-data() -> ("NewVal"=w247:dbl)  [unwired: 1 out]
        n147 = Divide(x=w247, y=100.0) -> (x/y=w246:dbl)
        n148 = Number To Fractional String(number=w246) -> (F-format string=w249:string)  [unwired: 3 in]
        n149 = Bundle By Name(cluster=w255, "Data Type"=Data_Types."Double", "Name"="HMI_TNK4_SuckPmpFrac_Setpoint", "Value"=w249) -> (w252:T1)
        n150 = Flatten To String(anything=w252) -> (data string=w251:string)  [unwired: 3 in, 2 out]
        n151 = call <vilib>:"Send Local Message.vi"("message queue in"=w256, "message name"="Write_Tag", "message value"=w251) -> ()  [unwired: 10 in, 3 out]
      }
      event Menu Selection (User) {
        # "Add run-time menu items to the message\nqueue. The message handler case names must match the menu ItemTag names."
        n152 = event-data() -> ("ItemTag"=w259:string)  [unwired: 1 out]
        n153 = call <vilib>:"Send Local Message.vi"("message queue in"=w258, "message name"=w259) -> ()  [unwired: 11 in, 3 out]
      }
      event "Cell T Last Hr": Value Change {
        n154 = event-data() -> ("NewVal"=w261:bool)  [unwired: 3 out]
        n155 = case shown="True" w261 {
          tunnel: w260 -> [_ w264]
          frame False {
          }
          frame True {
            n156 = call <vilib>:"Send Local Message.vi"("message queue in"=w264, "message name"="DisplayLastHr", "message value"="TNK4_Temperature") -> ()  [unwired: 10 in, 3 out]
          }
        }
      }
      event "BasT1_Level Last Hr": Value Change {
        n157 = event-data() -> ("NewVal"=w266:bool)  [unwired: 3 out]
        n158 = case shown="True" w266 {
          tunnel: w265 -> [_ w269]
          frame False {
          }
          frame True {
            n159 = call <vilib>:"Send Local Message.vi"("message queue in"=w269, "message name"="DisplayLastHr", "message value"="BAS_Proc2_Tank_Level") -> ()  [unwired: 10 in, 3 out]
          }
        }
      }
      event "BasT1_P Last Hr": Value Change {
        n160 = event-data() -> ("NewVal"=w271:bool)  [unwired: 3 out]
        n161 = case shown="True" w271 {
          tunnel: w270 -> [_ w274]
          frame False {
          }
          frame True {
            n162 = call <vilib>:"Send Local Message.vi"("message queue in"=w274, "message name"="DisplayLastHr", "message value"="TNK34_MainPressure") -> ()  [unwired: 10 in, 3 out]
          }
        }
      }
      event "MO": Value Change {
        n163 = event-data() -> ("NewVal"=w275:string)  [unwired: 6 out]
        n164 = shared-variable ".\\Local Variables.lvlib\\PT4_MO"(w275) -> ()  [unwired: 1 in, 1 out]
      }
      event "Rectifer Settings": Mouse Down {
        n165 = event-data() -> ("CtlRef"=w282:refnum<vi>, "Coords"=w280:T7, "Button"=w281:u16)  [unwired: 6 out]
        n166 = call "Handle Rectifer Step Selection.vi"("Coords"=w280, "Button"=w281, "MulticolumnListbox in"=w282) -> ("Row"=w278:i32)  [unwired: 8 in]
        n167 = Greater Than 0?(x=w278) -> (x > 0?=w279:bool)
        n168 = case shown="True" w279 {
          tunnel: w278 -> [_ w283]
          tunnel: w277 -> [_ w285]
          tunnel: w276 -> [_ w284]
          frame False {
          }
          frame True {
            n169 = Number To Decimal String(number=w283) -> (decimal integer string=w286:string)  [unwired: 1 in]
            n170 = Bundle By Name(cluster=w284, "Data Type"=Data_Types."I32", "Name"="HMI_Rect7_8_NumSteps", "Value"=w286) -> (w290:T1)
            n171 = Flatten To String(anything=w290) -> (data string=w289:string)  [unwired: 3 in, 2 out]
            n172 = call <vilib>:"Send Local Message.vi"("message queue in"=w285, "message name"="Write_Tag", "message value"=w289) -> ("message queue out"=w288:T5)  [unwired: 10 in, 2 out]
            n173 = call <vilib>:"Send Local Message.vi"("message queue in"=w288, "message name"="UpdatePlatingMinutes", "message value"=w286) -> ()  [unwired: 10 in, 3 out]
          }
        }
      }
      event "Rectifer Settings": Edit Cell {
        n174 = event-data() -> ("CtlRef"=w303:refnum<vi>, "String"=w301:string, "Coords"=w302:T8)  [unwired: 4 out]
        n175 = call "Data Check DC Rectifier Settings.vi"("String"=w301, "Coords"=w302, "MulticolumnListbox in"=w303) -> ("error out"=w298:errorcluster)  [unwired: 7 in, 1 out]
        n176 = shared-variable-read(refnum<k21> "ni.var.psp://z004551/CDL0100 ReadWriteTags/HMI_Rect7_8_NumSteps" ("shared variable refnum in"), 0) -> (w295:i32)  [unwired: 1 in, 3 out]
        n177 = Number To Decimal String(number=w295) -> (decimal integer string=w294:string)  [unwired: 1 in]
        n178 = call <vilib>:"Send Local Message.vi"("message queue in"=w299, "message name"="UpdatePlatingMinutes", "message value"=w294, "error in"=w298) -> ()  [unwired: 9 in, 3 out]
      }
    }
  }
  n179 = while "Message Processor" {
    shift-left: w2 -> [w313]
    shift-right: [w317] -> w8
    tunnel: w20 -> [w314]
    tunnel: w15 -> [w308]
    tunnel: [w308] -> w9
    shift-right: [w305] -> _
    shift-left: w7 -> [w306]
    tunnel: w1 -> [w304]
    stop <- w316 stop-if-true
    w309 = 100  # Timeout
    n180 = call <vilib>:"Read Next Message.vi"("message queue in"=w314, "timeout (1 ms)"=w309, "error in"=w313) -> ("exit process?"=w316:bool, "message queue out"=w315:T5, "message name"=w311:string, "message value"=w310:string, "error out"=w312:errorcluster)  [unwired: 5 in, 3 out]
    n181 = case shown="\"EZRecipe\"" w311 {
      selector: w311 -> [_ _ w409 _ _ _ _ _ _ _ _ _ _ _ _]
      tunnel: w315 -> [_ _ _ _ _ _ w499 _ _ _ _ w521 _ w548 w578]
      tunnel: w312 -> [w318 w330 w410 w411 w413 w415 w500 w502 w506 w509 w511 w524 w536 w541 w577]
      tunnel: [w318 w330 w410 errorcluster {"status"=FALSE, "code"=0, "source"=""} ("error out") w413 w415 w498 w502 w505 w509 w511 w518 w527 w545 w574] -> w317
      tunnel: w310 -> [_ _ _ _ _ _ _ _ w504 _ w513 w520 _ _ _]
      tunnel: w308 -> [_ _ _ _ _ _ _ _ w507 _ _ _ _ _ _]
      tunnel: T1 {"Data Type"=enum."Double", "Name"="test", "Value"="", "Description"=""} ("Tag") -> [_ _ _ _ _ _ _ _ _ _ _ _ _ _ _]
      tunnel: w306 -> [_ w325 _ _ _ w414 _ _ w503 w510 w512 _ w529 w549 w587]
      tunnel: [_ w326 _ _ _ w414 _ _ w503 w510 w512 _ w529 w549 w587] -> w305
      tunnel: w304 -> [_ _ _ _ _ _ _ _ _ _ _ _ _ w547 w576]
      frame "---------- Framework Operations ----------" {
        # "Dummy case to add a seperator in the Case Structure menu"
      }
      frame "", "Idle" {
        n182 = stacked-sequence {
          frame #0 {
            n183 = control-ref of="Enable Plating Cell"() -> (w336:refnum<vi>)
            n184 = shared-variable-read(refnum<k21> "ni.var.psp://z004551/CDL0100 ReadTags/Tnk4_Can_Plate" ("shared variable refnum in"), FALSE) -> (w346:bool)  [unwired: 1 in, 3 out]
            n185 = shared-variable-read(refnum<k21> "ni.var.psp://z004551/CDL0100 ReadWriteTags/HMI_Tank4_Enable" ("shared variable refnum in"), FALSE) -> (w333:bool)  [unwired: 1 in, 3 out]
            n186 = shared-variable-read(refnum<k21> "ni.var.psp://z004551/CDL0100 ReadWriteTags/HMI_Enable_BTnk2_Pump" ("shared variable refnum in"), FALSE) -> (w338:bool)  [unwired: 1 in, 3 out]
            n187 = shared-variable-read(refnum<k21> "ni.var.psp://z004551/CDL0100 ReadWriteTags/HMI_Tank3_Enable" ("shared variable refnum in"), FALSE) -> (w332:bool)  [unwired: 1 in, 3 out]
            n188 = Or(x=w333, y=w332) -> (x .or. y?=w331:bool)
            n189 = Or(x=w331, y=w338) -> (x .or. y?=w341:bool)
            n190 = case shown="False" w346 {
              tunnel: [T9."Disabled and Grayed Out" ("Disabled") T9."Enabled" ("Disabled")] -> w347
              frame False {
              }
              frame True {
              }
            }
            n191 = call "GrayOutButtonFromPSPVar.vi"("shared variable refnum in"=refnum<k21> "ni.var.psp://z004551/CDL0100 ReadWriteTags/HMI_Tank4_Drain", "Boolean in"=w336) -> ()  [unwired: 10 in]
            n192 = case shown="True" w341 {
              tunnel: [T9."Enabled" ("Disabled") T9."Disabled and Grayed Out" ("Disabled")] -> w340
              frame False {
              }
              frame True {
              }
            }
            n193 = control-ref of="Full Drain Plating Cell"() -> (w339:refnum<vi>)
            n194 = control-ref of="Start Cycle"() -> (w348:refnum<vi>)
            n195 = property class="Bool (strict)"(reference=w348, "DisabledEnum"=w347) -> ()  [unwired: 1 in, 2 out]
            n196 = property class="Bool (strict)"(reference=w339, "DisabledEnum"=w340) -> ()  [unwired: 1 in, 2 out]
          }
          frame #1 {
            n197 = shared-variable-read(refnum<k21> "ni.var.psp://z004551/CDL0100 ReadTags/IO_Bas_Tnk2_3Way_At_Recirc" ("shared variable refnum in"), FALSE) -> (w358:bool)  [unwired: 1 in, 3 out]
            n198 = shared-variable-read(refnum<k21> "ni.var.psp://z004551/CDL0100 ReadTags/IO_Bas_Tnk2_3Way_At_Open" ("shared variable refnum in"), FALSE) -> (w359:bool)  [unwired: 1 in, 3 out]
            n199 = shared-variable-read(refnum<k21> "ni.var.psp://z004551/CDL0100 ReadTags/IO_Bas_Tnk2_3Way_At_Closed" ("shared variable refnum in"), FALSE) -> (w362:bool)  [unwired: 1 in, 3 out]
            n200 = Or(x=w359, y=w358) -> (x .or. y?=w356:bool)
            "Sump Return" <- w356
            "Boolean 2" <- w356
            n201 = Or(x=w362, y=w359) -> (x .or. y?=w357:bool)
            "Return to sump" <- w357
            "Drain Tee Top" <- w357
            "Return to sump 2" <- w357
            "Process 1 Supply" <- w357
            n202 = Or(x=w357, y=w356) -> (x .or. y?=→"Boolean 5":bool)
          }
          frame #2 {
            n203 = shared-variable-read(refnum<k21> "ni.var.psp://z004551/CDL0100 ReadWriteTags/HMI_Tank4_Drain" ("shared variable refnum in"), FALSE) -> (w367:bool)  [unwired: 1 in, 3 out]
            n204 = shared-variable-read(refnum<k21> "ni.var.psp://z004551/CDL0100 ReadWriteTags/HMI_Enable_BTnk2_Pump" ("shared variable refnum in"), FALSE) -> (w368:bool)  [unwired: 1 in, 3 out]
            n205 = Or(x=w368, y=w367) -> (x .or. y?=→"SumpBottom":bool)
          }
          frame #3 {
            n206 = shared-variable-read(refnum<k21> "ni.var.psp://z004551/CDL0100 ReadTags/Rect7_8_CurrRecpStp" ("shared variable refnum in"), 0) -> (w374:i32)  [unwired: 1 in, 3 out]
            n207 = call-poly <userlib>:"Data Changed__ogtk.vi"("I32"=w374) -> ("Changed"=w375:bool)
            n208 = case shown="True" w375 {
              tunnel: w374 -> [_ w388]
              frame False {
              }
              frame True {
                w382 = 0.0 ("Scale.Range:Minimum")
                n209 = control-ref of="Left Anode Amp-min"() -> (w379:refnum<vi>)
                n210 = shared-variable-read(refnum<k21> "ni.var.psp://z004551/CDL0100 ReadWriteTags/HMI_Rct8_AMin_SetPnts" ("shared variable refnum in"), dbl[] []) -> (w383:dbl[])  [unwired: 1 in, 3 out]
                n211 = shared-variable-read(refnum<k21> "ni.var.psp://z004551/CDL0100 ReadWriteTags/HMI_Rect7_8_NumSteps" ("shared variable refnum in"), 0) -> (w389:i32)  [unwired: 1 in, 3 out]
                n212 = Less?(x=w388, y=w389) -> (x < y?=w390:bool)
                n213 = case shown="False" w390 {
                  tunnel: w388 -> [w396 w397]
                  tunnel: [w395 w397] -> w384
                  frame False {
                    n214 = Decrement(x=w396) -> (x-1=w395:i32)
                  }
                  frame True {
                  }
                }
                n215 = Index Array(array=w383, index=w384) -> (element=w380:dbl)
                n216 = control-ref of="Right Anode Amp-min"() -> (w378:refnum<vi>)
                n217 = shared-variable-read(refnum<k21> "ni.var.psp://z004551/CDL0100 ReadWriteTags/HMI_Rct7_AMin_SetPnts" ("shared variable refnum in"), dbl[] []) -> (w385:dbl[])  [unwired: 1 in, 3 out]
                n218 = Index Array(array=w385, index=w384) -> (element=w381:dbl)
                n219 = property class="Slide (strict)"(reference=w379, "Scale.Maximum"=w381, "Scale.Minimum"=w382) -> ()  [unwired: 1 in, 2 out]
                n220 = property class="Slide (strict)"(reference=w378, "Scale.Maximum"=w380, "Scale.Minimum"=w382) -> ()  [unwired: 1 in, 2 out]
              }
            }
          }
        }
        n221 = local read "Left Output On"() -> (w322:bool)
        n222 = local read "Right Output On"() -> (w323:bool)
        n223 = control-ref of="status"() -> (w329:refnum<vi>)
        n224 = Tick Count (ms)() -> (millisecond timer value=w324:u32)
        n225 = Subtract(x=w324, y=w325) -> (x-y=w327:u32)
        n226 = Or(x=w322, y=w323) -> (x .or. y?=w321:bool)
        n227 = call <userlib>:"TAE Format Alarm Ticker.vi"("Alarm Ticker Ref"=w329) -> ()  [unwired: 15 in]
        n228 = Greater?(x=w327, y=u32 500) -> (0:w320:bool)
        n229 = And(x=w321, y=w320) -> (x .and. y?=w319:bool)
        n230 = case shown="True" w319 {
          tunnel: w324 -> [_ w399]
          tunnel: [w398 w399] -> w326
          tunnel: w325 -> [w398 _]
          frame False {
          }
          frame True {
            n231 = shared-variable-read(refnum<k21> "ni.var.psp://z004551/CDL0100 ReadTags/Rect7_ActlVolts" ("shared variable refnum in"), 0.0) -> (w402:dbl)  [unwired: 1 in, 3 out]
            n232 = shared-variable-read(refnum<k21> "ni.var.psp://z004551/CDL0100 ReadTags/Rect8_ActlVolts" ("shared variable refnum in"), 0.0) -> (w401:dbl)  [unwired: 1 in, 3 out]
            n233 = Bundle(w402, w401) -> (→"Output Voltage":cluster{dbl, dbl})  [unwired: 1 in]
          }
        }
      }
      frame "Missing Message Handler", Default {
        # "Call this case if a message is received that is not handled \nby any other case. Typically this is a programming error\nas a result of a typo or unhandled message/missing message handler."
        n234 = Format Into String(format string="DevError: Missing message handler for '%s\" message." ("message"), w409) -> (resulting string=w407:string)  [unwired: 2 in, 1 out]
        n235 = One Button Dialog(message=w407) -> ()  [unwired: 2 out]
      }
      frame "Error" {
        # "General Error Case - this case is called if an error is passed using the error cluster below. Typically most new errors should be handed in each individual case and not passed in the rror cluster. If necessary a custom error handler case should be added and called from other cases."
        n236 = call <vilib>:"Simple Error Handler.vi"("error in (no error)"=w411) -> ()  [unwired: 1 in, 8 out]
      }
      frame "---------- Generic Operations ----------" {
        # "Dummy case to add a seperator in the Case Structure menu"
      }
      frame "Initialize" {
        n237 = stacked-sequence {
          seq-local: [_ _ w451 _ _] -> [_ _ _ w471 w478]
          seq-local: [_ _ w448 _ _] -> [_ _ _ w469 w483]
          seq-local: [_ _ w447 _ _] -> [_ _ _ w467 w482]
          frame #0 {
            n238 = shared-variable-read(refnum<k21> "ni.var.psp://z004551/CDL0100 ReadWriteTags/HMI_TNK4_SuckPmpFrac_Setpoint" ("shared variable refnum in"), 0.0) -> (w418:dbl)  [unwired: 1 in, 3 out]
            n239 = shared-variable-read(refnum<k21> "ni.var.psp://z004551/CDL0100 ReadWriteTags/HMI_Tnk4_Enable_SuckPump" ("shared variable refnum in"), FALSE) -> (w421:bool)  [unwired: 1 in, 3 out]
            n240 = shared-variable-read(refnum<k21> "ni.var.psp://z004551/CDL0100 ReadWriteTags/HMI_Tnk3_Rack_RPM" ("shared variable refnum in"), 0.0) -> (w432:dbl)  [unwired: 1 in, 3 out]
            n241 = shared-variable-read(refnum<k21> "ni.var.psp://z004551/CDL0100 ReadWriteTags/HMI_Tank4_Rack_Motor_Run" ("shared variable refnum in"), FALSE) -> (w431:bool)  [unwired: 1 in, 3 out]
            n242 = shared-variable-read(refnum<k21> "ni.var.psp://z004551/CDL0100 ReadWriteTags/HMI_TNK4_Flow_Setpoint" ("shared variable refnum in"), 0.0) -> (w430:dbl)  [unwired: 1 in, 3 out]
            n243 = Multiply(x=w418, y=100.0) -> (x*y=w416:dbl)
            n244 = local write "Enable Suck Pump"(w421) -> ()
            n245 = local write "Rack RPM"(w432) -> ()
            n246 = local write "Enable Rack Motion"(w431) -> ()
            n247 = local write "Total Inflow (L/min)"(w430) -> ()
            n248 = local write "Suck Pump fraction of inflow"(w416) -> ()
          }
          frame #1 {
            n249 = shared-variable-read(refnum<k21> "ni.var.psp://z004551/CDL0100 ReadWriteTags/HMI_Tank4_Drain" ("shared variable refnum in"), FALSE) -> (w433:bool)  [unwired: 1 in, 3 out]
            n250 = shared-variable-read(refnum<k21> "ni.var.psp://z004551/CDL0100 ReadWriteTags/HMI_Tnk3_Eductor_RPM" ("shared variable refnum in"), 0.0) -> (w441:dbl)  [unwired: 1 in, 3 out]
            n251 = shared-variable-read(refnum<k21> "ni.var.psp://z004551/CDL0100 ReadWriteTags/HMI_Tank4_Enable" ("shared variable refnum in"), FALSE) -> (w440:bool)  [unwired: 1 in, 3 out]
            n252 = local write "Full Drain Plating Cell"(w433) -> ()
            n253 = shared-variable-read(refnum<k21> "ni.var.psp://z004551/CDL0100 ReadWriteTags/HMI_Tank4_Eductor_Motors_Run" ("shared variable refnum in"), FALSE) -> (w444:bool)  [unwired: 1 in, 3 out]
            n254 = local write "Enable Plating Cell"(w440) -> ()
            n255 = local write "Eductor RPM"(w441) -> ()
            n256 = local write "Enable Eductor Motion"(w444) -> ()
          }
          frame #2 {
            w449 = 0.0
            n257 = shared-variable ".\\Local Variables.lvlib\\PT4_MO"() -> (w445:string)  [unwired: 1 in, 1 out]
            n258 = shared-variable-read(refnum<k21> "ni.var.psp://z004551/CDL0100 ReadWriteTags/HMI_Rct7_AMin_SetPnts" ("shared variable refnum in"), dbl[] []) -> (w448:dbl[])  [unwired: 1 in, 3 out]
            n259 = shared-variable-read(refnum<k21> "ni.var.psp://z004551/CDL0100 ReadWriteTags/HMI_Rect5_6_NumSteps" ("shared variable refnum in"), 0) -> (w451:i32)  [unwired: 1 in, 3 out]
            n260 = shared-variable-read(refnum<k21> "ni.var.psp://z004551/CDL0100 ReadWriteTags/HMI_BAS_TNK2_P_Setpoint" ("shared variable refnum in"), 0.0) -> (w458:dbl)  [unwired: 1 in, 3 out]
            n261 = shared-variable-read(refnum<k21> "ni.var.psp://z004551/CDL0100 ReadWriteTags/HMI_Rct8_AMin_SetPnts" ("shared variable refnum in"), dbl[] []) -> (w447:dbl[])  [unwired: 1 in, 3 out]
            n262 = local write "Supply Pressure (kPa)"(w458) -> ()
            n263 = for {
              N: w451 -> [_]
              tunnel: w448 -> [w466] mode=indexing
              shift-right: [w464] -> w450
              shift-left: w449 -> [w465]
              n264 = Add(x=w466, y=w465) -> (x+y=w464:dbl)
            }
            n265 = for {
              tunnel: w447 -> [w463] mode=indexing
              shift-right: [w461] -> w446
              shift-left: w449 -> [w462]
              n266 = Add(x=w463, y=w462) -> (x+y=w461:dbl)
            }
            n267 = local write "Total Amp*min L"(w450) -> ()
            n268 = local write "MO"(w445) -> ()
            n269 = local write "Total Amp*min R"(w446) -> ()
          }
          frame #3 {
            n270 = control-ref of="Rectifer Settings"() -> (w472:refnum<vi>)
            n271 = shared-variable-read(refnum<k21> "ni.var.psp://z004551/CDL0100 ReadWriteTags/HMI_Rct7_A_SetPnts" ("shared variable refnum in"), dbl[] []) -> (w470:dbl[])  [unwired: 1 in, 3 out]
            n272 = shared-variable-read(refnum<k21> "ni.var.psp://z004551/CDL0100 ReadWriteTags/HMI_Rct8_A_SetPnts" ("shared variable refnum in"), dbl[] []) -> (w468:dbl[])  [unwired: 1 in, 3 out]
            n273 = call "Write Rectifier Recipe to ListBox.vi"("Right AmpMins"=w467, "Left AmpMins"=w469, "Right Amps"=w468, "Left Amps"=w470, "Number Steps"=w471, "ListBox"=w472) -> ()  [unwired: 5 in, 1 out]
          }
          frame #4 {
            n274 = control-ref of="Rectifer Settings"() -> (w494:refnum<vi>)
            n275 = control-ref of="Left Anode Amp-min"() -> (w480:refnum<vi>)
            n276 = control-ref of="Right Anode Amp-min"() -> (w481:refnum<vi>)
            n277 = property class="MCListbox (strict)"(reference=w494) -> ("ItemNames"=w493:string[][])  [unwired: 1 in, 2 out]
            n278 = call "Calculate Plating Time DC.vi"("ItemNames"=w493, "Num Steps"=w478) -> ("Right Anode Time"=w489:dbl, "Left Anode Time"=w490:dbl)  [unwired: 8 in]
            n279 = shared-variable-read(refnum<k21> "ni.var.psp://z004551/CDL0100 ReadTags/Rect5_6_CurrRecpStp" ("shared variable refnum in"), 0) -> (w477:i32)  [unwired: 1 in, 3 out]
            n280 = Less?(x=w477, y=w478) -> (x < y?=w488:bool)
            n281 = local write "Right Time"(w489) -> ()
            n282 = local write "Left Time"(w490) -> ()
            n283 = case shown="False" w488 {
              tunnel: w477 -> [w496 w497]
              tunnel: [w495 w497] -> w479
              frame False {
                n284 = Decrement(x=w496) -> (x-1=w495:i32)
              }
              frame True {
              }
            }
            n285 = Index Array(array=w483, index=w479) -> (element=w487:dbl)
            n286 = Index Array(array=w482, index=w479) -> (element=w484:dbl)
            n287 = property class="Slide (strict)"(reference=w480, "Scale.Maximum"=w487, "Scale.Minimum"=0.0 ("Scale.Range:Minimum")) -> ()  [unwired: 1 in, 2 out]
            n288 = property class="Slide (strict)"(reference=w481, "Scale.Maximum"=w484, "Scale.Minimum"=0.0 ("Scale.Range:Minimum")) -> ()  [unwired: 1 in, 2 out]
          }
        }
      }
      frame "Exit" {
        # "Destroy message queue >> this will halt the UI event handler loop"
        # "Stop the VI\n>> Perform any cleanup tasks in this message case.\n>> Clear display before closing."
        n289 = call <vilib>:"Destroy Message Queue.vi"("message queue in"=w499, "error in"=w500) -> ("error out"=w498:errorcluster)  [unwired: 11 in, 2 out]
        n290 = local write "status"("" ("Status")) -> ()
      }
      frame "---------- Application Operations ----------" {
        # "Dummy case to add a seperator in the Case Structure menu"
      }
      frame "Write_Tag" {
        n291 = call-poly <vilib>:"Write Message.vi"("error in"=w506, "data"=w504, "name"="WriteTag", "connection info in"=w507) -> ("error out"=w505:errorcluster)  [unwired: 6 in, 1 out]
      }
      frame "UpdateVPlotX" {
      }
      frame "DisplayLastHr" {
        n292 = call "Trace Variable 1 hour Popup.vi"("Tag"=w513) -> ()  [unwired: 11 in]
      }
      frame "UpdatePlatingMinutes" {
        n293 = control-ref of="Rectifer Settings"() -> (w522:refnum<vi>)
        n294 = Decimal String To Number(string=w520) -> (number=w519:i32)  [unwired: 2 in, 1 out]
        n295 = call "Assemble DC Rectifier Setting Changes for PLC.vi"("Num Steps"=w519, "Rect Number"=7, "error In"=w524, "message queue in"=w521, "MulticolumnListbox in"=w522) -> ("Right Anode Mins"=w514:dbl, "Left Anode Mins"=w516:dbl, "Right AmpMin"=w515:dbl, "Left AmpMin"=w517:dbl, "error out"=w518:errorcluster)  [unwired: 2 in]
        n296 = local write "Total Amp*min L"(w517) -> ()
        n297 = local write "Total Amp*min R"(w515) -> ()
        n298 = local write "Right Time"(w514) -> ()
        n299 = local write "Left Time"(w516) -> ()
      }
      frame "Save_Recipe" {
        n300 = control-ref of="Rectifer Settings"() -> (w537:refnum<vi>)
        n301 = call "Convert DC RectifierListData to Arrays.vi"("error in (no error)"=w536, "MulticolumnListbox in"=w537) -> ("error out"=w535:errorcluster, "Right Amps"=w533:dbl[], "Left Amps"=w534:dbl[], "Right Amp Min"=w531:dbl[], "Left AmpMins"=w532:dbl[])  [unwired: 5 in]
        n302 = shared-variable-read(refnum<k21> "ni.var.psp://z004551/CDL0100 ReadWriteTags/HMI_Rect7_8_NumSteps" ("shared variable refnum in"), 0) -> (w530:i32)  [unwired: 1 in, 3 out]
        n303 = call "Save Rectifier Recipe.vi"("Rev Mult"=0.0, "Right AmpMins"=w531, "Left AmpMins"=w532, "error in"=w535, "Number Steps"=w530, "Right Amps"=w533, "Left Amps"=w534) -> ("error out"=w527:errorcluster, "name"=w525:string, "cancelled"=w526:bool)  [unwired: 2 in]
        n304 = case shown="False" w526 {
          tunnel: w525 -> [w540 _]
          frame False {
            n305 = local write "Loaded Recipe"(w540) -> ()
          }
          frame True {
          }
        }
      }
      frame "Load_A_Recipe" {
        n306 = control-ref of="Rectifer Settings"() -> (w546:refnum<vi>)
        n307 = call "BrowseRecipe.vi"("error in (no error)"=w541) -> ("error out"=w542:errorcluster, "cancelled"=w543:bool, "selected path"=w544:path)  [unwired: 8 in]
        n308 = case shown="False" w543 {
          tunnel: w542 -> [w554 w573]
          tunnel: [w551 w573] -> w545
          tunnel: w548 -> [w564 _]
          tunnel: w547 -> [w563 _]
          tunnel: w544 -> [w553 _]
          tunnel: w546 -> [w552 _]
          frame False {
            n309 = call "Read Rectifier Recipe.vi"("selected path"=w553, "error in"=w554) -> ("Left Amps"=w560:dbl[], "Left AmpMins"=w559:dbl[], "Num Steps"=w558:i32, "name"=w550:string, "Right Amps"=w557:dbl[], "Right AmpMins"=w556:dbl[], "error out"=w555:errorcluster)  [unwired: 5 in, 2 out]
            n310 = local write "Loaded Recipe"(w550) -> ()
            n311 = call "Write Rectifier Recipe to ListBox.vi"("Right AmpMins"=w556, "Left AmpMins"=w559, "Right Amps"=w557, "Left Amps"=w560, "error in (no error)"=w555, "Number Steps"=w558, "ListBox"=w552) -> ("error out"=w562:errorcluster)  [unwired: 4 in]
            n312 = Number To Decimal String(number=w558) -> (decimal integer string=w565:string)  [unwired: 1 in]
            n313 = Bundle By Name(cluster=w563, "Data Type"=Data_Types."I32", "Name"="HMI_Rect7_8_NumSteps", "Value"=w565) -> (w569:T1)
            n314 = Flatten To String(anything=w569) -> (data string=w568:string)  [unwired: 3 in, 2 out]
            n315 = call <vilib>:"Send Local Message.vi"("message queue in"=w564, "message name"="Write_Tag", "message value"=w568, "error in"=w562) -> ("message queue out"=w567:T5, "error out"=w561:errorcluster)  [unwired: 9 in, 1 out]
            n316 = call <vilib>:"Send Local Message.vi"("message queue in"=w567, "message name"="UpdatePlatingMinutes", "message value"=w565, "error in"=w561) -> ("error out"=w551:errorcluster)  [unwired: 9 in, 2 out]
          }
          frame True {
          }
        }
      }
      frame "EZRecipe" {
        w586 = T10 7 items=["User Home"=0, "User Desktop"=1, "User Documents"=2, "User Application Data"=3, "User Preferences"=4, "User Temporary"=5, "Public Documents"=6, "Public Application Data"=7, "Public Preferences"=8, "Public Cache"=13, "System Core Libraries"=9, "System Installed Libraries"=10, "Application Files"=11, "Boot Volume Root"=12] ("system directory type")
        n317 = control-ref of="Rectifer Settings"() -> (w575:refnum<vi>)
        n318 = local read "Loaded Recipe"() -> (w581:string)
        n319 = call <vilib>:"Get System Directory.vi"("system directory type"=w586) -> ("system directory"=w583:path)  [unwired: 10 in]
        n320 = Build Path(base path=w583, name or relative path="TDK\\CDL0100") -> (appended path=w584:path)
        n321 = Build Path(base path=w584, name or relative path=w581) -> (appended path=w582:path)
        n322 = call "CDL0100 Recipe Creator v1.1.vi"("Previous Recipe Path"=w582) -> ("New Recipe Path"=w580:path, "canceled?"=w579:bool)  [unwired: 1 out]
        n323 = case shown="False" w579 {
          tunnel: w577 -> [w592 w611]
          tunnel: [w589 w611] -> w574
          tunnel: w578 -> [w602 _]
          tunnel: w576 -> [w601 _]
          tunnel: w580 -> [w591 _]
          tunnel: w575 -> [w590 _]
          frame False {
            n324 = call "Read Rectifier Recipe.vi"("selected path"=w591, "error in"=w592) -> ("Left Amps"=w598:dbl[], "Left AmpMins"=w597:dbl[], "Num Steps"=w596:i32, "name"=w588:string, "Right Amps"=w595:dbl[], "Right AmpMins"=w594:dbl[], "error out"=w593:errorcluster)  [unwired: 5 in, 2 out]
            n325 = local write "Loaded Recipe"(w588) -> ()
            n326 = call "Write Rectifier Recipe to ListBox.vi"("Right AmpMins"=w594, "Left AmpMins"=w597, "Right Amps"=w595, "Left Amps"=w598, "error in (no error)"=w593, "Number Steps"=w596, "ListBox"=w590) -> ("error out"=w600:errorcluster)  [unwired: 4 in]
            n327 = Number To Decimal String(number=w596) -> (decimal integer string=w603:string)  [unwired: 1 in]
            n328 = Bundle By Name(cluster=w601, "Data Type"=Data_Types."I32", "Name"="HMI_Rect7_8_NumSteps", "Value"=w603) -> (w607:T1)
            n329 = Flatten To String(anything=w607) -> (data string=w606:string)  [unwired: 3 in, 2 out]
            n330 = call <vilib>:"Send Local Message.vi"("message queue in"=w602, "message name"="Write_Tag", "message value"=w606, "error in"=w600) -> ("message queue out"=w605:T5, "error out"=w599:errorcluster)  [unwired: 9 in, 1 out]
            n331 = call <vilib>:"Send Local Message.vi"("message queue in"=w605, "message name"="UpdatePlatingMinutes", "message value"=w603, "error in"=w599) -> ("error out"=w589:errorcluster)  [unwired: 9 in, 2 out]
          }
          frame True {
          }
        }
      }
    }
  }
  n332 = call-poly <vilib>:"Get Connection Reference.vi"("error in"=w8, "connection info in"=w9) -> ("error out"=w12:errorcluster, "connection ID out"=w11:refnum<k5>)  [unwired: 8 out]
  n333 = TCP Close Connection(connection ID=w11, error in (no error)=w12) -> (error out=w14:errorcluster)  [unwired: 2 out]
  n334 = call <vilib>:"Error to Warning.vi"("1st Error to Convert"=w13, "error in"=w14) -> ("warning out"=w10:errorcluster)  [unwired: 3 in, 10 out]
  n335 = call <vilib>:"Simple Error Handler.vi"("error in (no error)"=w10) -> ()  [unwired: 4 in, 5 out]
